vi "TDK_InitCom.vi"(8 "error in (no error)":errorcluster, 11 "VISA name":refnum<visa-resource-name>) -> (0 "error out":errorcluster, 3 "VISA name":refnum<visa-resource-name>)   [LabVIEW 2015]
uses:
  <vilib>/Instr/_visa.llb/VISA Configure Serial Port (Serial Instr).vi
panel:
  in  "General Settings:Timeout Value":u32=2000
  in  "flow control (0:none)":u16(ring)=1 caption="流控制（0:无）" items=["无", "XON/XOFF", "RTS/CTS", "XON/XOFF & RTS/CTS", "DTR/DSR", "XON/XOFF & DTR/DSR"]
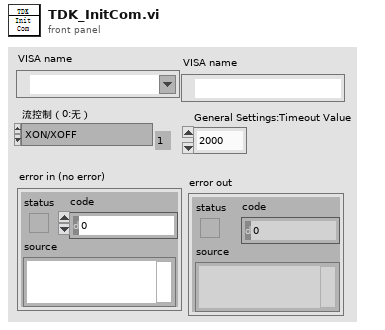
[diagram p1: front panel]
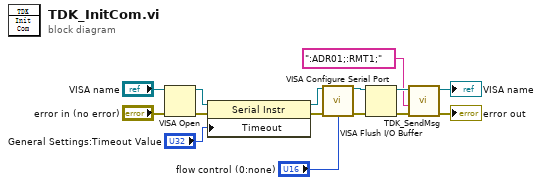
[diagram p0: block diagram]
diagram:
  n1 = VISA Open(error in (no error)="error in (no error)", VISA resource name="VISA name") -> (VISA resource name=w12:refnum<visa-resource-name>, error out=w10:errorcluster)  [unwired: 3 in]
  n2 = property class="Serial Instr"(reference=w12, error in=w10, "Timeout"="General Settings:Timeout Value") -> (reference out=w11:refnum<visa-resource-name>, error out=w9:errorcluster)
  n3 = call-poly "VISA Configure Serial Port"("VISA resource name"=w11, "error in (no error)"=w9, "flow control (0:none)"="flow control (0:none)") -> ("VISA resource name out"=w13:refnum<visa-resource-name>, "error out"=w14:errorcluster)  [unwired: 11 in]
  n4 = VISA Flush I/O Buffer(VISA resource name=w13, error in (no error)=w14) -> (VISA resource name out=w8:refnum<visa-resource-name>, error out=w7:errorcluster)  [unwired: 1 in]
  n5 = call "TDK_SendMsg.vi"("error in (no error)"=w7, "CMD"=":ADR01;:RMT1;" ("Command Out"), "VISA resource name"=w8) -> ("error out"=→"error out":errorcluster, "VISA resource name"=→"VISA name":refnum<visa-resource-name>)  [unwired: 3 in, 2 out]
